vi "Clear test data.vi"   [LabVIEW 2009]
uses:
  Global 1.vi
types:
  T1 = cluster{"People":string, "product  number":string, "Test time":string, "VHeatFuse_noload":string, "VHeatFuse_load":string, "VoverrideDiode":string, "Test firmware upload via X1":string, "TemperAddress":string, "Troom":string, "TLCU":string, "Adjustment factor":string, "MeasuredFreq":string, "I2C communication":string, "Light-emitting diode on Z2":string, "Battery warning/inhibit":string, "Reset by IC10":string, "External EEPROM":string, "RFID card detection and reading RFID":string, "Production parameters in internal EEPROM":string, "Current consumption in sleep mode":string, "Application and database upload":string, "Test result":string, "Table head[22]":string, "Table head[23]":string}
  T2 = cluster{"serial number":string, "Part number":string, "Revision letter ":string, "Revision counter":string, "Manufature":string, "Year Week":string}
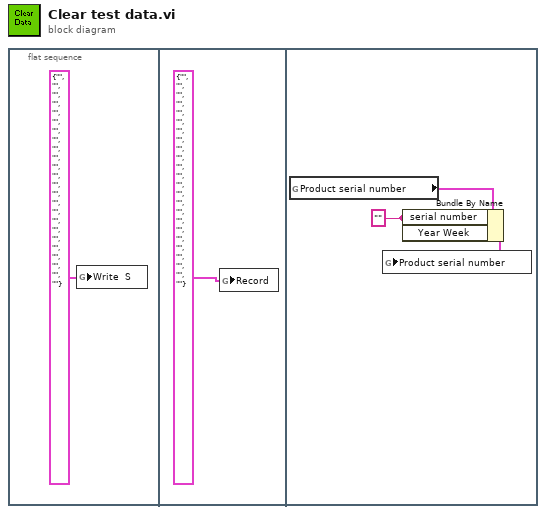
[diagram p0: block diagram]
diagram:
  n1 = flat-sequence {
    frame #0 {
      n2 = global write "Global 1.vi" "Write  S"(T1 {"People"="", "product  number"="", "Test time"="", "VHeatFuse_noload"="", "VHeatFuse_load"="", "VoverrideDiode"="", "Test firmware upload via X1"="", "TemperAddress"="", "Troom"="", "TLCU"="", "Adjustment factor"="", "MeasuredFreq"="", "I2C communication"="", "Light-emitting diode on Z2"="", "Battery warning/inhibit"="", "Reset by IC10"="", "External EEPROM"="", "RFID card detection and reading RFID"="", "Production parameters in internal EEPROM"="", "Current consumption in sleep mode"="", "Application and database upload"="", "Test result"="", "Table head[22]"="", "Table head[23]"=""} ("Write  S")) -> ()
    }
    frame #1 {
      n3 = global write "Global 1.vi" "Record"(T1 {"People"="", "product  number"="", "Test time"="", "VHeatFuse_noload"="", "VHeatFuse_load"="", "VoverrideDiode"="", "Test firmware upload via X1"="", "TemperAddress"="", "Troom"="", "TLCU"="", "Adjustment factor"="", "MeasuredFreq"="", "I2C communication"="", "Light-emitting diode on Z2"="", "Battery warning/inhibit"="", "Reset by IC10"="", "External EEPROM"="", "RFID card detection and reading RFID"="", "Production parameters in internal EEPROM"="", "Current consumption in sleep mode"="", "Application and database upload"="", "Test result"="", "Table head[22]"="", "Table head[23]"=""} ("Record")) -> ()
    }
    frame #2 {
      w4 = "" ("serial number")
      n4 = global read "Global 1.vi" "Product serial number"() -> (w3:T2)
      n5 = Bundle By Name(cluster=w3, "serial number"=w4, "Year Week"=w4) -> (w5:T2)
      n6 = global write "Global 1.vi" "Product serial number"(w5) -> ()
    }
  }
